vi "James and Nathan Fail.vi"(10 "Dashboard Ops":T1[](array[typedef])) -> (2 "Output":string[](array[string]))   [LabVIEW 2012]
uses:
  AutoInstruction.ctl
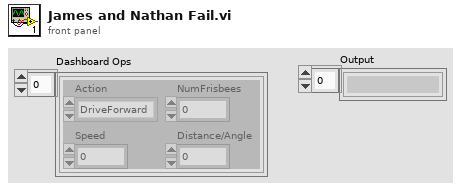
[diagram p1: front panel]
types:
  T1 = typedef "AutoInstruction.ctl" = cluster{"Distance/Angle":dbl, "Speed":dbl, "Action":enum16{"DriveForward", "Turn", "Aim", "Shoot"}, "NumFrisbees":i32}
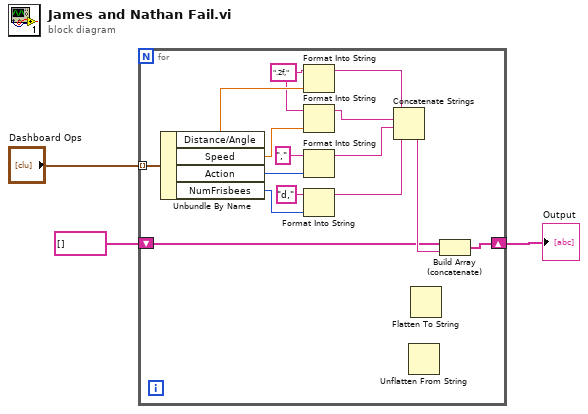
[diagram p0: block diagram]
diagram:
  n1 = for {
    tunnel: "Dashboard Ops" -> [w18] mode=indexing
    shift-right: [w5] -> w1
    shift-left: string[] [] ("Array") -> [w4]
    w13 = ".2f,"
    n2 = Unbundle By Name(w18) -> ("Distance/Angle"=w14:dbl, "Speed"=w15:dbl, "Action"=w16:enum16{"DriveForward", "Turn", "Aim", "Shoot"}, "NumFrisbees"=w17:i32)
    n3 = Format Into String(initial string=w13, w14) -> (resulting string=w10:string)  [unwired: 2 in, 1 out]
    n4 = Format Into String(initial string=w13, w15) -> (resulting string=w9:string)  [unwired: 2 in, 1 out]
    n5 = Format Into String(initial string=",", w16) -> (resulting string=w8:string)  [unwired: 2 in, 1 out]
    n6 = Format Into String(initial string="d,", w17) -> (resulting string=w7:string)  [unwired: 2 in, 1 out]
    n7 = Concatenate Strings(w10, w9, w8, w7) -> (w6:string)
    n8 = Unflatten From String() -> ()  [unwired: 5 in, 3 out]
    n9 = Flatten To String() -> ()  [unwired: 4 in, 3 out]
    n10 = Build Array (concatenate)(w4, w6) -> (w5:string[])
  }
  "Output" <- w1
